vi "ChiStrategy.vi"(9 "ChiChoice":u16[][](array[ring]), 10 "Hand":u16[](array[ring])) -> (2 "Result":i16)   [LabVIEW 2025]
panel:
  out "HandCount":u16[](array[numeric])
  out "Max":i16
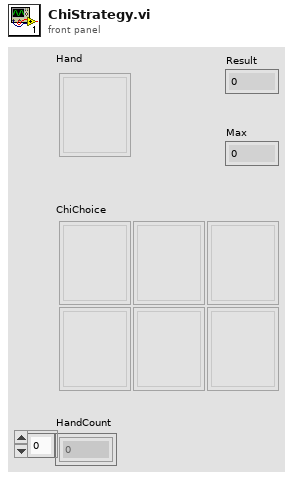
[diagram p1: front panel]
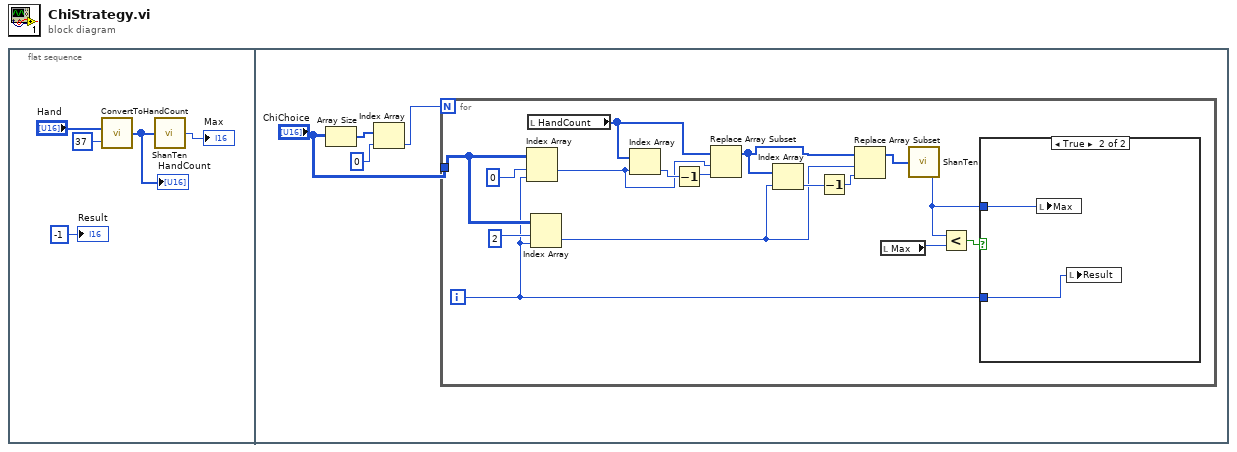
[diagram p0: block diagram]
diagram:
  n1 = flat-sequence {
    frame #0 {
      n2 = call "ConvertToHandCount.vi"("AddtionalTile"=u16 37, "Hand"="Hand") -> ("HandCount"=w1:u16[])
      "HandCount" <- w1
      n3 = call "ShanTen.vi"("Count"=w1) -> ("ShanTen"=→"Max":i16)
      "Result" <- i16 -1 ("Result")
    }
    frame #1 {
      n4 = Array Size(array="ChiChoice") -> (size(s)=w9:i32[])
      n5 = Index Array(array=w9, index=0) -> (element=w8:i32)
      n6 = for {
        N: w8 -> [_]
        tunnel: "ChiChoice" -> [w24]
        i -> [w10]
        n7 = Index Array(array=w24, index (row)=0, index (col)=w10) -> (element=w19:u16)
        n8 = local read "HandCount"() -> (w22:u16[])
        n9 = Index Array(array=w24, index (row)=2, index (col)=w10) -> (element=w15:u16)
        n10 = Index Array(array=w22, index=w19) -> (element=w20:u16)
        n11 = Decrement(x=w20) -> (x-1=w21:u16)
        n12 = Replace Array Subset(array=w22, new element=w21, index=w19) -> (w18:u16[])
        n13 = Index Array(array=w18, index=w15) -> (element=w16:u16)
        n14 = Decrement(x=w16) -> (x-1=w17:u16)
        n15 = Replace Array Subset(array=w18, new element=w17, index=w15) -> (w14:u16[])
        n16 = local read "Max"() -> (w12:i16)
        n17 = call "ShanTen.vi"("Count"=w14) -> ("ShanTen"=w11:i16)
        n18 = Less?(x=w11, y=w12) -> (x < y?=w13:bool)
        n19 = case shown="True" w13 {
          tunnel: w11 -> [_ w27]
          tunnel: w10 -> [_ w26]
          frame False {
          }
          frame True {
            n20 = local write "Max"(w27) -> ()
            n21 = local write "Result"(w26) -> ()
          }
        }
      }
    }
  }
